vi "Constants.vi"() -> ()   [LabVIEW 2016, in "Untitled Project 1 Shared.lvlib"]
doc: "Use this Global VI to access the GUIDs assigned to the page resources of the Custom Device."
uses:
  Untitled Project 1 Shared.lvlib
panel:
  in  "Tab Control":enum32{"GUIDS", "Constants", "Properties"}(tab)
  in  "Untitled Project 1":string="76019636-9dee-4b93-a964-7cfadac394e7"
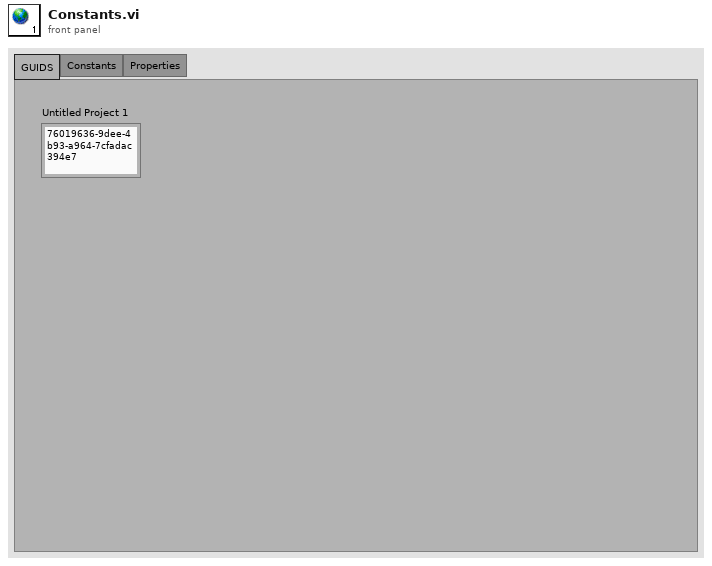
[diagram p1: front panel]
diagram:
